vi "SVI_CheckAndIncrementFilename.vi"(0 "selected path":path) -> (1 "Filename":string, 2 "File Path":path)   [LabVIEW 2014]
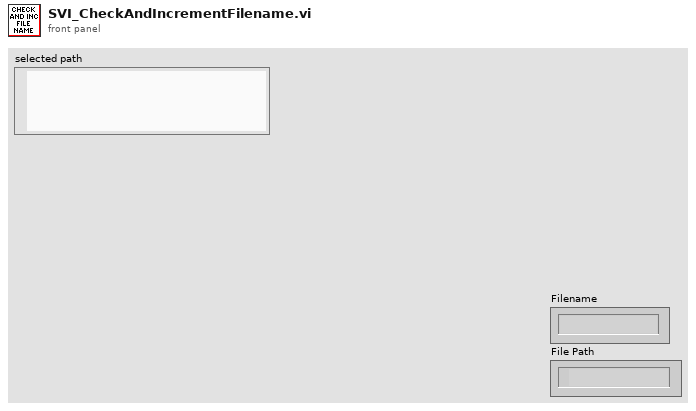
[diagram p1: front panel]
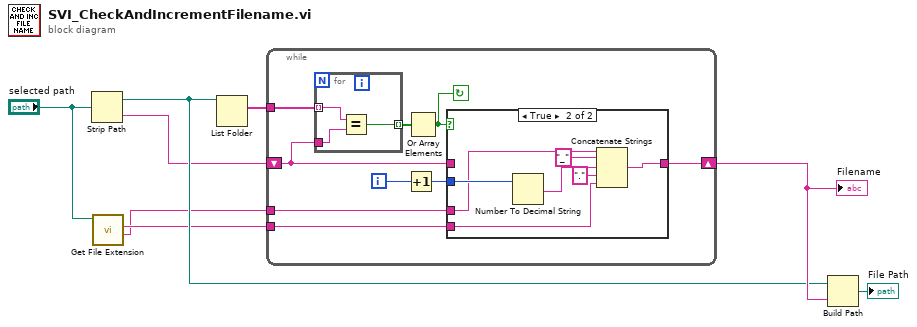
[diagram p0: block diagram]
diagram:
  n1 = Strip Path(path="selected path") -> (stripped path=w5:path, name=w2:string)
  n2 = call <vilib>:"Get File Extension.vi"("file"="selected path") -> ("filename without extension"=w1:string, "lowercase file extension"=w3:string)  [unwired: 7 in, 2 out]
  n3 = List Folder(path=w5) -> (filenames=w8:string[])  [unwired: 3 in, 3 out]
  n4 = while {
    tunnel: w8 -> [w17]
    shift-right: [w14] -> w7
    shift-left: w2 -> [w15]
    tunnel: w1 -> [w10]
    tunnel: w3 -> [w9]
    i -> [w12]
    stop <- w13 continue-if-true
    n5 = for {
      tunnel: w17 -> [w28] mode=indexing
      tunnel: w15 -> [w27]
      tunnel: [w26] -> w16 mode=indexing
      n6 = Equal?(x=w28, y=w27) -> (x = y?=w26:bool)
    }
    n7 = Increment(x=w12) -> (x+1=w11:i32)
    n8 = Or Array Elements(Boolean array=w16) -> (logical OR=w13:bool)
    n9 = case shown="True" w13 {
      tunnel: w15 -> [w18 _]
      tunnel: [w18 w23] -> w14
      tunnel: w11 -> [_ w25]
      tunnel: w10 -> [_ w24]
      tunnel: w9 -> [_ w19]
      frame False {
      }
      frame True {
        n10 = Number To Decimal String(number=w25) -> (decimal integer string=w22:string)  [unwired: 1 in]
        n11 = Concatenate Strings(w24, "_" ("string"), w22, "." ("string"), w19) -> (w23:string)
      }
    }
  }
  "Filename" <- w7
  n12 = Build Path(base path=w5, name or relative path=w7) -> (appended path=→"File Path":path)
